vi "MKS946_Main.vi"(7 "stop_external":refnum<vi>, 8 "input cluster":T1) -> (4 "error out":errorcluster={"status"=FALSE, "code"=0, "source"="0"})   [LabVIEW 2019]
doc: "Perform the acquisition. Replace the contents of this diagram with calls to acquisition hardware.\n_____\nBased on Delacor QMH Project Template 5.0.0.82."
uses:
  cluster_ref_MKS946.ctl
panel:
  out "Status":bool
  in  "n_pt_max":i32=100 caption="in plot"
  in  "interval":dbl=0.5 caption="in sec" format="%#_13g"
  out "graph_ch2":T2(graph)
  out "graph_ch1":T2(graph)
  in  "stop":bool
  out "P2":dbl
  out "P1":dbl
  out "measurement time":timestamp format="%<%H:%M:%S\n%Y/%m/%d>T"
  in  "address":i32=253
  out "visa_out":refnum<visa-resource-name>
  in  "visa_in":refnum<visa-resource-name>="COM14"
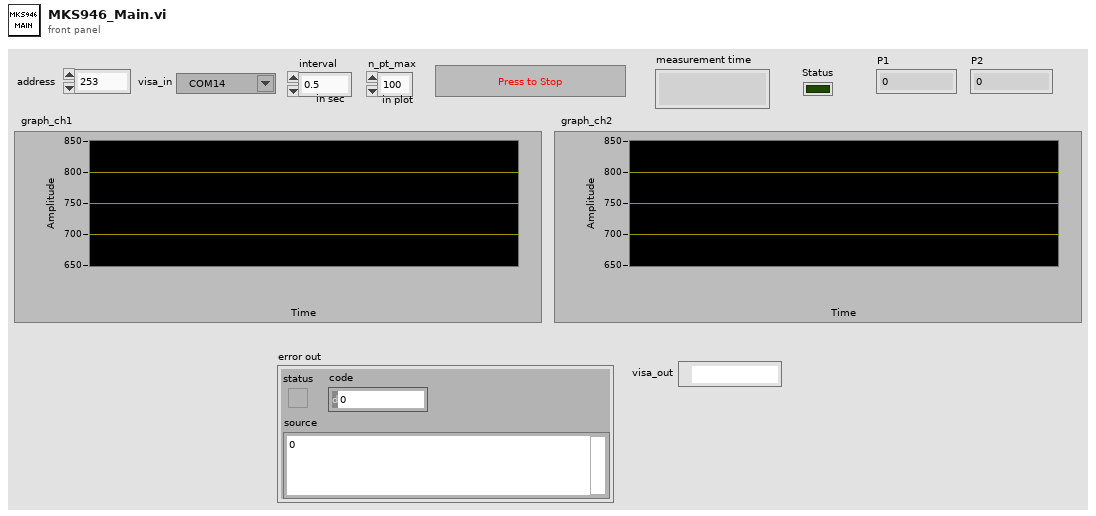
[diagram p1: front panel]
types:
  T1 = typedef "cluster_ref_MKS946.ctl" = cluster{"Status":refnum<vi>, "PR1":refnum<vi>, "PR2":refnum<vi>}
  T2 = cluster{"seconds since 1Jan1904":timestamp, "value":dbl}[]
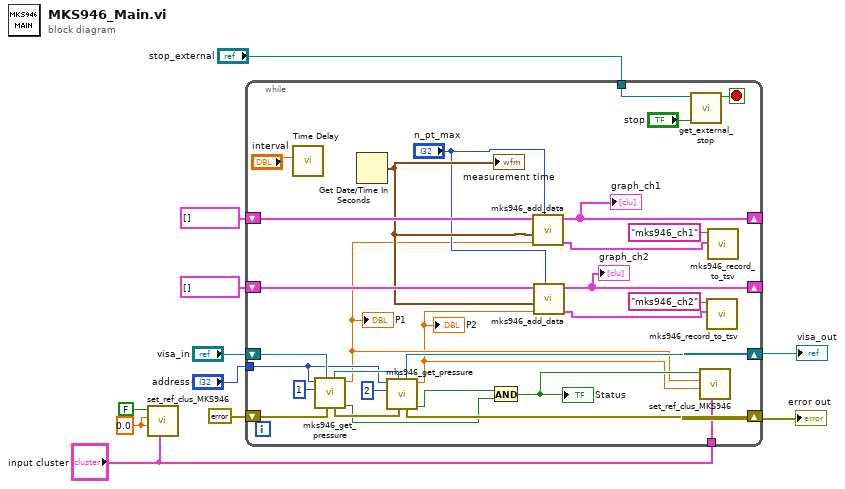
[diagram p0: block diagram]
diagram:
  w1 = 0.0 ("PR2")
  n1 = call "set_ref_clus_MKS946.vi"("cluster_ref"="input cluster", "PR2"=w1, "PR1"=w1, "status"=FALSE) -> ()  [unwired: 8 in]
  n2 = while {
    tunnel: "address" -> [w33]
    shift-right: [w36] -> w9
    shift-left: "visa_in" -> [w40]
    shift-right: [w32] -> w7
    shift-left: errorcluster {"status"=FALSE, "code"=0, "source"=""} ("error in") -> [w38]
    shift-right: [w27] -> _
    shift-left: T2 [] ("graph_ch1") -> [w28]
    shift-right: [w25] -> _
    shift-left: T2 [] ("graph_ch1") -> [w24]
    tunnel: "input cluster" -> [w12]
    tunnel: "stop_external" -> [w15]
    stop <- w13 stop-if-true
    n3 = call "Time Delay"("Delay Time (s)"="interval") -> ()  [unwired: 10 in, 1 out]
    n4 = call "mks946_get_pressure.vi"("err_in"=w38, "visa_in"=w40, "channel"=1, "address"=w33) -> ("status"=w19:bool, "value"=w17:dbl, "err_out"=w35:errorcluster, "visa_out"=w37:refnum<visa-resource-name>)  [unwired: 3 in, 1 out]
    "P1" <- w17
    n5 = Get Date/Time In Seconds() -> (seconds since 1Jan1904=w23:timestamp)
    "measurement time" <- w23
    n6 = call "mks946_get_pressure.vi"("err_in"=w35, "visa_in"=w37, "channel"=2, "address"=w33) -> ("status"=w20:bool, "value"=w16:dbl, "err_out"=w32:errorcluster, "visa_out"=w36:refnum<visa-resource-name>)  [unwired: 3 in, 1 out]
    "P2" <- w16
    n7 = And(x=w20, y=w19) -> (x .and. y?=w18:bool)
    "Status" <- w18
    n8 = call "mks946_add_data.vi"("n_max"="n_pt_max", "value"=w17, "timestamp"=w23, "array_in"=w28) -> ("cluster_out"=w26:cluster{"timestamp":timestamp, "value":dbl}, "array_out"=w27:T2)  [unwired: 6 in]
    "graph_ch1" <- w27
    n9 = call "mks946_add_data.vi"("n_max"="n_pt_max", "value"=w16, "timestamp"=w23, "array_in"=w24) -> ("cluster_out"=w22:cluster{"timestamp":timestamp, "value":dbl}, "array_out"=w25:T2)  [unwired: 6 in]
    "graph_ch2" <- w25
    n10 = call "get_external_stop.vi"("stop_internal"="stop", "ref_stop_external"=w15) -> ("stop_output"=w13:bool)  [unwired: 9 in]
    n11 = call "set_ref_clus_MKS946.vi"("cluster_ref"=w12, "PR2"=w16, "PR1"=w17, "status"=w18) -> ()  [unwired: 8 in]
    n12 = call "mks946_record_to_tsv.vi"("cluster"=w22, "name"="mks946_ch2") -> ()  [unwired: 10 in]
    n13 = call "mks946_record_to_tsv.vi"("cluster"=w26, "name"="mks946_ch1") -> ()  [unwired: 10 in]
  }
  "error out" <- w7
  "visa_out" <- w9
